vi "readPressureTransducers.vi"(8 "error in":errorcluster) -> (0 "error out":errorcluster, 2 "Analog Pressure Reading":T1)   [LabVIEW 2017]
uses:
  Type Defs/AnalogPressureReading.ctl
  <vilib>/myRIO/Instrument Drivers/Onboard IO/AI/typedefs/AI Reference.ctl
  <vilib>/myRIO/Common/Instrument Driver Framework/Utilities/typedefs/myRIO Generic Hardware Reference.ctl
  <vilib>/myRIO/Common/Instrument Driver Framework/Utilities/typedefs/Hardware Version Enum.ctl
  <vilib>/myRIO/Common/Instrument Driver Framework/Utilities/typedefs/myRIO v1.0 Reference.ctl
  <vilib>/myRIO/Common/Instrument Driver Framework/Utilities/typedefs/Generic FPGA Reference.ctl
  <vilib>/myRIO/Common/Instrument Driver Framework/myRIO v1.0/AI/typedefs/AI Channels List.ctl
  <vilib>/myRIO/Common/Instrument Driver Framework/myRIO v1.0/AI/typedefs/AI Channels Enum.ctl
  <vilib>/myRIO/Common/Instrument Driver Framework/Utilities/typedefs/Analog Scaling Constants List.ctl
  <vilib>/myRIO/Common/Instrument Driver Framework/Utilities/typedefs/Analog Scaling Constants.ctl
  <vilib>/userdefined/High Color/nirio_resource_hc.ctl
  <vilib>/myRIO/Common/Instrument Driver Framework/Utilities/vis/Is FPGA Ref Available.vi
  <vilib>/myRIO/Common/Instrument Driver Framework/myRIO v1.0/AI/vis/myRIO v1.1 Open AI.vi
  <vilib>/myRIO/Instrument Drivers/Onboard IO/AI/vis/Read.vi
  <vilib>/myRIO/Common/Instrument Driver Framework/Utilities/vis/Validate Channels.vi
  <vilib>/myRIO/Common/Instrument Driver Framework/myRIO v1.0/AI/vis/myRIO v1.0 Reserve AI.vi
  <vilib>/myRIO/Common/Instrument Driver Framework/myRIO v1.0/AI/vis/myRIO v1.0 Build MUX Configuration AI.vi
  <vilib>/myRIO/Common/Instrument Driver Framework/myRIO v1.0/Resource Manager/vis/myRIO v1.0 Reserve Channel List.vi
  <vilib>/myRIO/Common/Instrument Driver Framework/myRIO v1.0/Resource Manager/vis/myRIO v1.0 Reserve Channel.vi
  <vilib>/myRIO/Common/Instrument Driver Framework/myRIO v1.0/Resource Manager/vis/myRIO v1.0 Unreserve Channel.vi
  <vilib>/myRIO/Common/Instrument Driver Framework/myRIO v1.0/Resource Manager/vis/myRIO v1.0 Build Mutex Name.vi
  <vilib>/Utility/VariantDataType/GetNumericInfo.vi
  <vilib>/Utility/error.llb/Error Cluster From Error Code.vi
  <vilib>/myRIO/Common/Instrument Driver Framework/myRIO v1.0/myRIO v1.1 Open.vi
  <vilib>/myRIO/Common/Instrument Driver Framework/myRIO v1.0/AI/vis/myRIO v1.0 Get Scaling Constants AI.vi
  <vilib>/myRIO/Common/Instrument Driver Framework/Utilities/vis/IO Manager.vi
  <vilib>/myRIO/Common/Instrument Driver Framework/Utilities/vis/Configuration Manager.vi
  <vilib>/myRIO/Common/Instrument Driver Framework/myRIO v1.0/myRIO v1.0 Close.vi
  <vilib>/myRIO/Common/Instrument Driver Framework/myRIO v1.0/AI/vis/myRIO v1.0 Read AI.vi
  <vilib>/myRIO/Express VI/Onboard IO/AI/AI Express VI.xnode
  <vilib>/myRIO/Instrument Drivers/Onboard IO/AI/vis/myRIO AI Open.xnode
  <vilib>/myRIO/Instrument Drivers/Onboard IO/AI/AI.lvlib
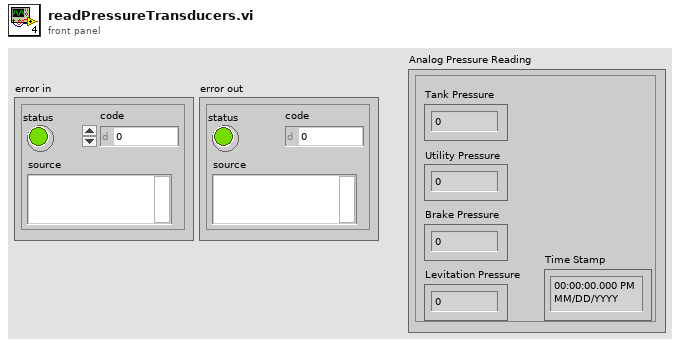
[diagram p1: front panel]
types:
  T1 = typedef "AnalogPressureReading.ctl" = cluster{"Tank Pressure":dbl, "Utility Pressure":dbl, "Brake Pressure":dbl, "Levitation Pressure":dbl, "Time Stamp":timestamp}
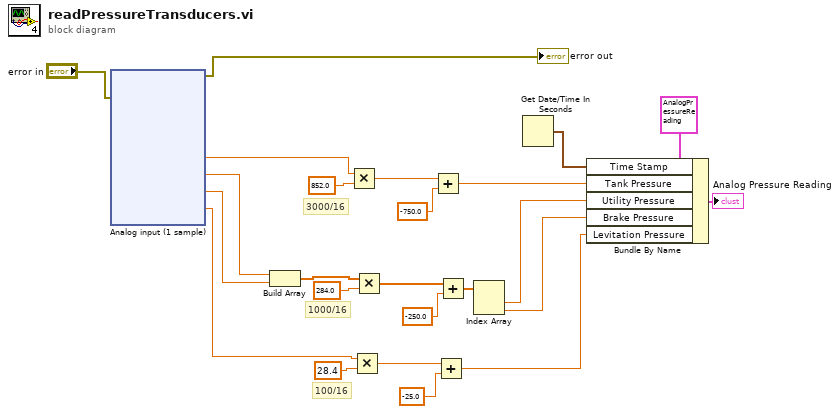
[diagram p0: block diagram]
diagram:
  # "100/16"
  # "1000/16"
  # "3000/16"
  n1 = xnode "Analog input (1 sample)"("error in (no error)"="error in") -> ("A/AI0 (Pin 3)"=w8:dbl, "A/AI1 (Pin 5)"=w10:dbl, "A/AI2 (Pin 7)"=w9:dbl, "A/AI3 (Pin 9)"=w7:dbl, "error out"=→"error out":errorcluster)
  n2 = Build Array(w10, w9) -> (w6:dbl[])
  n3 = Multiply(x=w8, y=852.0 ("A/AI2 (Pin 7)")) -> (x*y=w22:dbl)
  n4 = Multiply(x=w7, y=28.4 ("A/AI2 (Pin 7)")) -> (x*y=w12:dbl)
  n5 = Multiply(x=w6, y=284.0 ("A/AI2 (Pin 7)")) -> (x*y=w15:dbl[])
  n6 = Add(x=w22, y=-750.0 ("A/AI2 (Pin 7)")) -> (x+y=w4:dbl)
  n7 = Add(x=w12, y=-25.0 ("A/AI2 (Pin 7)")) -> (x+y=w1:dbl)
  n8 = Add(x=w15, y=-250.0 ("A/AI2 (Pin 7)")) -> (x+y=w5:dbl[])
  n9 = Index Array(array=w5) -> (element #1=w3:dbl, element #2=w2:dbl)  [unwired: 2 in]
  n10 = Get Date/Time In Seconds() -> (seconds since 1Jan1904=w17:timestamp)
  n11 = Bundle By Name(cluster=T1 {"Tank Pressure"=0.0, "Utility Pressure"=0.0, "Brake Pressure"=0.0, "Levitation Pressure"=0.0, "Time Stamp"=timestamp(0 s since 1904-01-01)} ("Analog Pressure Reading"), "Time Stamp"=w17, "Tank Pressure"=w4, "Utility Pressure"=w3, "Brake Pressure"=w2, "Levitation Pressure"=w1) -> (→"Analog Pressure Reading":T1)
